vi "Message filter.vi"(6 "module state":T1, 9 "response notifier in":refnum<notifier>, 10 "message in":string) -> (3 "msg out":string)   [LabVIEW 2019, in "Communication Interface.lvlib"]
uses:
  Communication Interface.lvlib
  module state.ctl
  Intertarget communication/Status + response + data cluster.ctl
  Intertarget communication/CommandResponse communication.lvlib
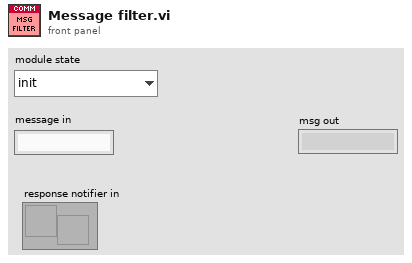
[diagram p1: front panel]
types:
  T1 = typedef "Communication Interface.lvlib/module state.ctl" = enum16{"init", "wait on connection", "communication", "close"}
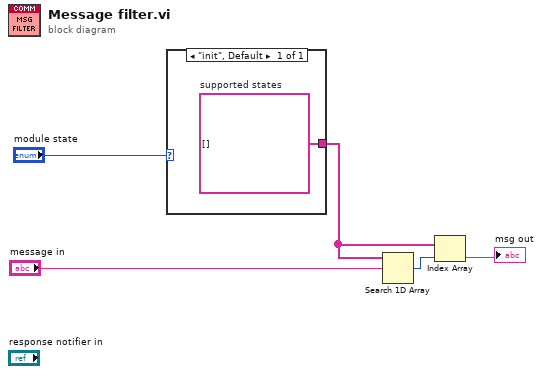
[diagram p0: block diagram]
diagram:
  n1 = case shown="\"init\", Default" "module state" {
    tunnel: [w6] -> w2
    frame "init", Default {
      w6 = string[] []  # supported states
    }
  }
  n2 = Search 1D Array(1D array=w2, element="message in") -> (index of element=w3:i32)  [unwired: 1 in]
  n3 = Index Array(array=w2, index=w3) -> (element=→"msg out":string)
